vi "ReadDID_ReturnASCII.vi"(8 "error in (no error)":errorcluster, 10 "ID":u16, 11 "Ref":T1) -> (0 "error out":errorcluster, 2 "Raw ASCII":string, 3 "Ref":T1)   [LabVIEW 2019, in "Diagnostics Host Automation API.lvlib"]
uses:
  Shared/Types/HostAutomation.Ref.ctl
  <vilib>/NI/STM/TCP/TCP Connection Info.ctl
  <vilib>/NI/STM/SubVIs/MetaDataElement.ctl
  Shared/Types/DTC.Codes.ctl
  Engine/Types/Frame.Data.ctl
  Diagnostics Host Automation API.lvlib
  <vilib>/NI/NIVS Addon Network Comm/Shared/NI VeriStand Addon Network Comm Shared.lvlib
  Engine/Diagnostics Addon Engine.lvlib
  <vilib>/NI/STM/NI STM.lvlib
  Shared/Diagnostics Addon Shared.lvlib
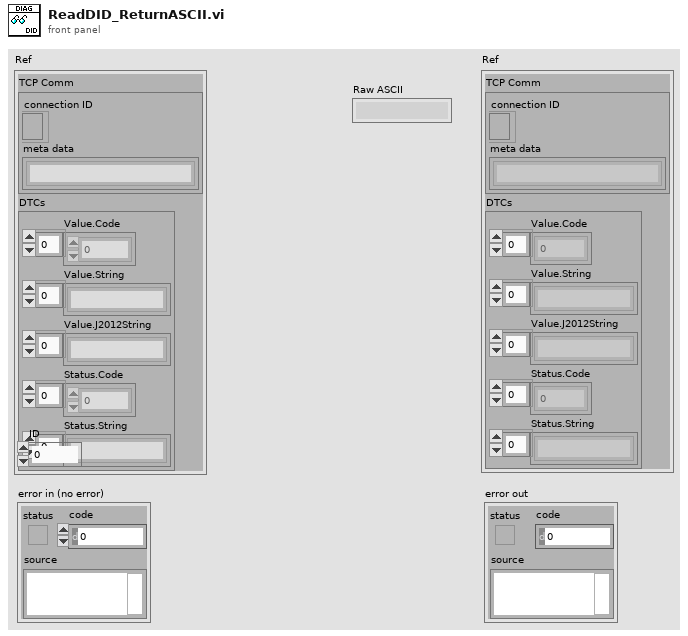
[diagram p1: front panel]
types:
  T1 = typedef "Diagnostics Addon Shared.lvlib/HostAutomation.Ref.ctl" = cluster{"TCP Comm":T2, "DTCs":T4}
  T2 = typedef "NI STM.lvlib/TCP Connection Info.ctl" = cluster{"connection ID":refnum<k5>, "meta data":T3[]}
  T3 = typedef "NI STM.lvlib/MetaDataElement.ctl" = string
  T4 = typedef "Diagnostics Addon Shared.lvlib/DTC.Codes.ctl" = cluster{"Value.Code":dbl[], "Value.String":string[], "Value.J2012String":string[], "Status.Code":dbl[], "Status.String":string[]}
  T5 = typedef "Diagnostics Addon Engine.lvlib/Frame.Data.ctl" = cluster{"ID":u32, "Raw Frame":u8[]}
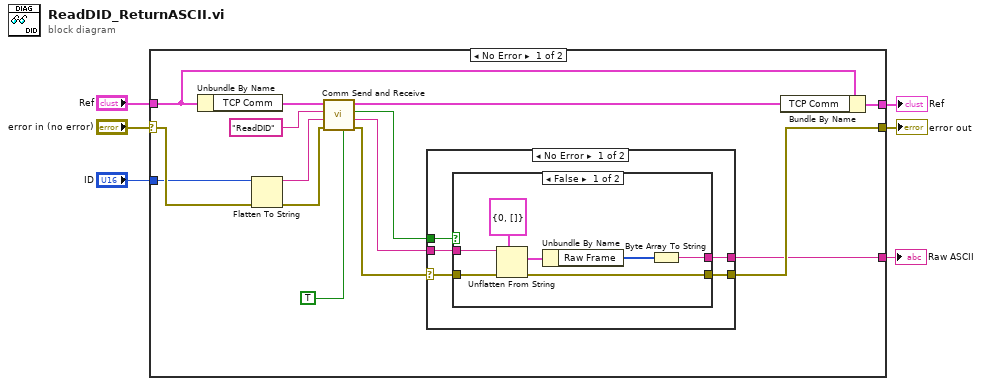
[diagram p0: block diagram]
diagram:
  n1 = case shown="No Error" "error in (no error)" {
    selector: "error in (no error)" -> [w19 w37]
    tunnel: "Ref" -> [w15 w36]
    tunnel: [w13 w36] -> w5
    tunnel: [w9 w37] -> w4
    tunnel: "ID" -> [w17 _]
    tunnel: [w8 _] -> w1
    frame No Error {
      n2 = Unbundle By Name(w15) -> ("TCP Comm"=w16:T2)
      n3 = Flatten To String(anything=w17, error in (no error)=w19) -> (data string=w20:string, error out=w18:errorcluster)  [unwired: 2 in, 1 out]
      n4 = call <vilib>:"Comm Send and Receive.vi"("Resp Required?"=TRUE, "error in (no error)"=w18, "Data"=w20, "Name"="ReadDID", "connection info"=w16) -> ("error out"=w10:errorcluster, "Data"=w12:string, "Timed Out?"=w11:bool, "connection info"=w14:T2)  [unwired: 3 in]
      n5 = case shown="No Error" w10 {
        selector: w10 -> [w24 w35]
        tunnel: w11 -> [w26 _]
        tunnel: [w25 w35] -> w9
        tunnel: w12 -> [w23 _]
        tunnel: [w22 _] -> w8
        frame No Error {
          n6 = case shown="False" w26 {
            tunnel: [w32 w34] -> w25
            tunnel: w24 -> [w33 w34]
            tunnel: w23 -> [w31 _]
            tunnel: [w27 _] -> w22
            frame False {
              n7 = Unflatten From String(type=T5 {"ID"=0, "Raw Frame"=[]} ("cluster"), binary string=w31, error in (no error)=w33) -> (value=w29:T5, error out=w32:errorcluster)  [unwired: 2 in, 1 out]
              n8 = Unbundle By Name(w29) -> ("Raw Frame"=w28:u8[])
              n9 = Byte Array To String(unsigned byte array=w28) -> (string=w27:string)
            }
            frame True {
            }
          }
        }
        frame Error {
        }
      }
      n10 = Bundle By Name(cluster=w15, "TCP Comm"=w14) -> (w13:T1)
    }
    frame Error {
    }
  }
  "Ref" <- w5
  "error out" <- w4
  "Raw ASCII" <- w1
